vi "Result.Attribute, Convert EV1 to EV2 Format.vi"(11 "Attr EV1":T1[](array[typedef]) {"Status" items=["LOG", "PASS", "FAIL", "ERROR"]}) -> (3 "Attr EV2":T3[](array[typedef]) {"Status" items=["LOG", "PASS", "FAIL", "ERROR"]})   [LabVIEW 2019]
uses:
  Result.Attribute.ctl
  Result.Measurement and Attribute Item Status.ctl
  Result.Attribute_EV1.ctl
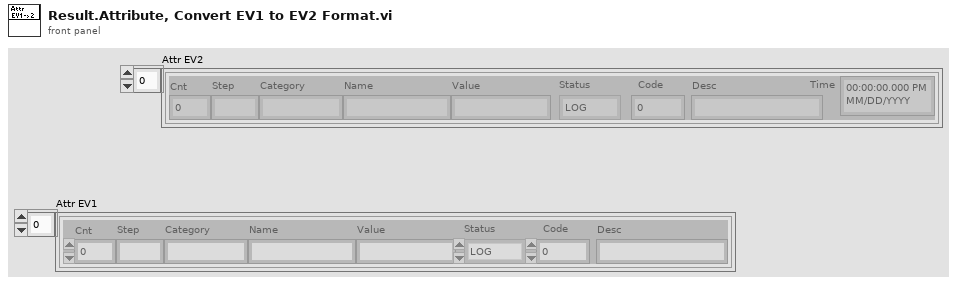
[diagram p1: front panel]
types:
  T1 = typedef "Result.Attribute_EV1.ctl" = cluster{"Cnt":i32, "Step":string, "Category":string, "Name":string, "Value":string, "Status":T2, "Code":i32, "Desc":string}
  T2 = typedef "Result.Measurement and Attribute Item Status.ctl" = i32
  T3 = typedef "Result.Attribute.ctl" = cluster{"Cnt":i32, "Step":string, "Category":string, "Name":string, "Value":string, "Status":T2, "Code":i32, "Desc":string, "Time":timestamp}
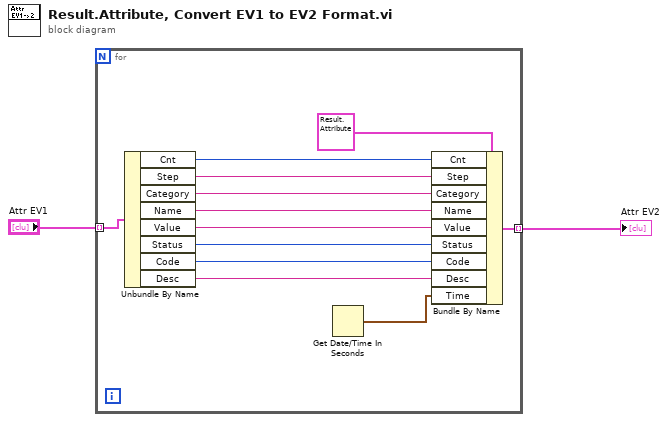
[diagram p0: block diagram]
diagram:
  n1 = for {
    tunnel: "Attr EV1" -> [w14] mode=indexing
    tunnel: [w13] -> w1 mode=indexing
    n2 = Unbundle By Name(w14) -> ("Cnt"=w12:i32, "Step"=w11:string, "Category"=w10:string, "Name"=w9:string, "Value"=w8:string, "Status"=w7:T2, "Code"=w6:i32, "Desc"=w5:string)
    n3 = Get Date/Time In Seconds() -> (seconds since 1Jan1904=w3:timestamp)
    n4 = Bundle By Name(cluster=T3 {"Cnt"=0, "Step"="", "Category"="", "Name"="", "Value"="", "Status"=0, "Code"=0, "Desc"="", "Time"=timestamp(0 s since 1904-01-01)} ("Attribute"), "Cnt"=w12, "Step"=w11, "Category"=w10, "Name"=w9, "Value"=w8, "Status"=w7, "Code"=w6, "Desc"=w5, "Time"=w3) -> (w13:T3)
  }
  "Attr EV2" <- w1
